vi "Example Callback - Illuminance Callback.vi"(4 "Illuminance":refnum<user-event>, 5 "Event Data":cluster{"sender":refnum<k24>, "illuminance":i32}, 6 "Control Ref":refnum<k24>, 7 "Event Common Data":T1) -> ()   [LabVIEW 2013]
uses:
  C:/tf/play/labview/Tinkerforge.dll
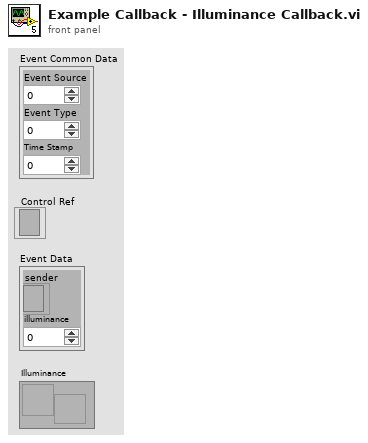
[diagram p1: front panel]
types:
  T1 = cluster{"Event Source":i32, "Event Type":u32, "Time Stamp":u32}
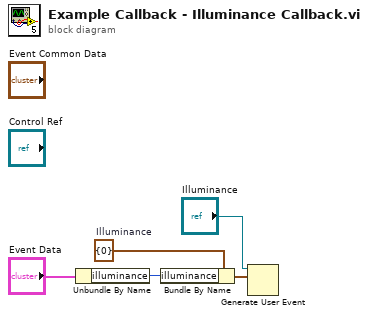
[diagram p0: block diagram]
diagram:
  w3 = cluster{"illuminance":i32} {"illuminance"=0}  # Illuminance
  n1 = Unbundle By Name("Event Data") -> ("illuminance"=w2:i32)
  n2 = Bundle By Name(cluster=w3, "illuminance"=w2) -> (w1:cluster{"illuminance":i32})
  n3 = Generate User Event(user event="Illuminance", event data cluster=w1) -> ()  [unwired: 2 in, 2 out]
